vi "WPI_SerialPortGetBytesReceived.vi"(8 "error in (no error)":errorcluster, 11 "SerialPortRef":T1) -> (0 "error out":errorcluster, 2 "Bytes at Port":u32, 3 "SerialPortRef":T1)   [LabVIEW 2017]
doc: "Returns the number of bytes in the input buffer of the serial device you specify.\n\nThis software is licensed. Open the labview\\readme\\WPI Robotics Library Open Source License.txt file for more information."
uses:
  <vilib>/Rock Robotics/WPI/SerialPort/WPI_SerialPortRef.ctl
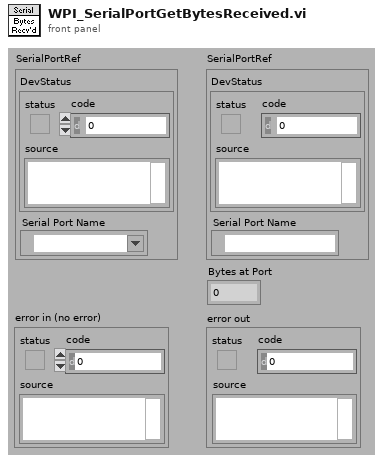
[diagram p1: front panel]
types:
  T1 = typedef "WPI_SerialPortRef.ctl" = cluster{"DevStatus":errorcluster, "Serial Port Name":refnum<visa-resource-name>}
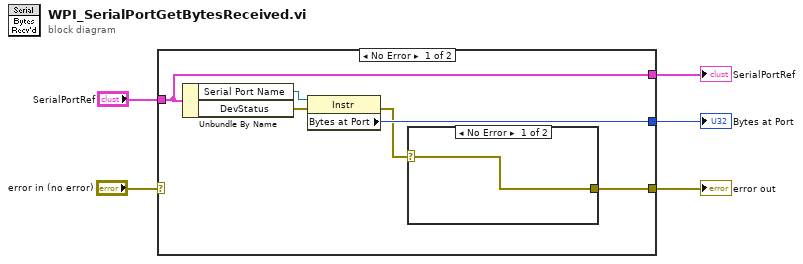
[diagram p0: block diagram]
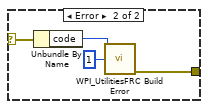
[diagram p2: hidden frame]
diagram:
  n1 = case shown="No Error" "error in (no error)" {
    selector: "error in (no error)" -> [_ w18]
    tunnel: "SerialPortRef" -> [w6 w17]
    tunnel: [w6 w17] -> w4
    tunnel: [w7 w18] -> w2
    tunnel: [w9 _] -> w1
    frame No Error {
      n2 = Unbundle By Name(w6) -> ("Serial Port Name"=w11:refnum<visa-resource-name>, "DevStatus"=w10:errorcluster)
      n3 = property class="Instr"(reference=w11, error in=w10) -> (error out=w8:errorcluster, "Bytes at Port"=w9:u32)  [unwired: 1 in]
      n4 = case shown="No Error" w8 {
        selector: w8 -> [w12 w14]
        tunnel: [w12 w13] -> w7
        frame No Error {
        }
        frame Error {
          n5 = Unbundle By Name(w14) -> ("code"=w16:i32)
          n6 = call <vilib>:"WPI_UtilitiesFRC Build Error.vi"("error code"=w16, "chain levels to remove (1)"=1) -> ("error out"=w13:errorcluster)  [unwired: 3 in, 10 out]
        }
      }
    }
    frame Error {
    }
  }
  "error out" <- w2
  "SerialPortRef" <- w4
  "Bytes at Port" <- w1
